vi "load config data.vi"(8 "error in (no error)":errorcluster, 11 "Sim Laser Driver in":refnum<class "Sim Laser Driver.lvclass">) -> (0 "error out":errorcluster, 3 "Sim Laser Driver out":refnum<class "Sim Laser Driver.lvclass">)   [LabVIEW 2022 SP3, in "Sim Laser Driver.lvclass"]
uses:
  Sim Laser Driver.lvclass
  C:/XY Stage/XY Stage/Framework/Base/Base.lvclass
  XY Stage/Framework/Base/Base.lvclass/Base.ctl
  Sim Laser Driver.lvclass/Sim Laser Driver.ctl
  c45f4fda-8063-4fab-8851-1de7a636a2c7.vi
  XY Stage/Framework/Base/Accessors/Read Config Path.vi
  XY Stage/Framework/Base/Accessors/Read Section.vi
  <vilib>/Utility/config.llb/Open Config Data.vi
  <userlib>/_OpenG.lib/variantconfig/variantconfig.llb/Read Section Cluster__ogtk.vi
  <vilib>/Utility/config.llb/Close Config Data.vi
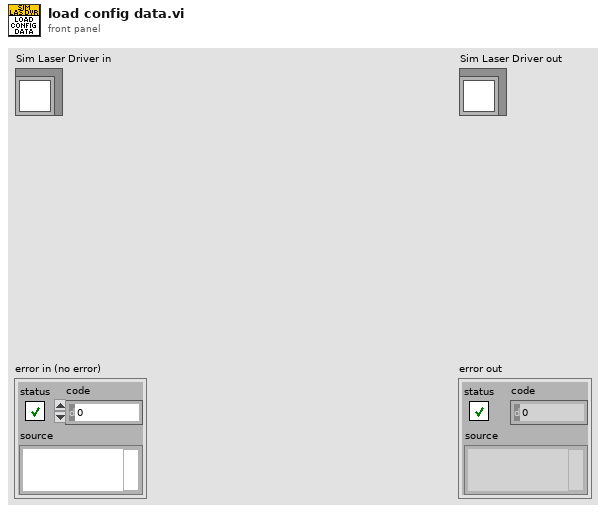
[diagram p1: front panel]
types:
  T1 = typedef "Sim Laser Driver.lvclass/settings.ctl" = cluster{"Power":dbl}
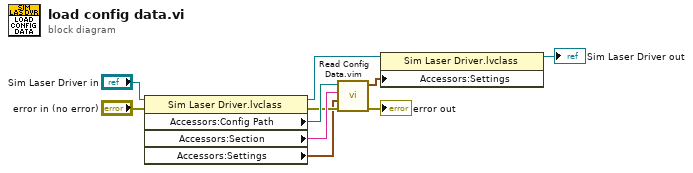
[diagram p0: block diagram]
diagram:
  n1 = property class="Sim Laser Driver.lvclass"(reference="Sim Laser Driver in", error in="error in (no error)") -> (reference out=w3:refnum<class "Sim Laser Driver.lvclass">, error out=w8:errorcluster, "Accessors:Config Path"=w10:path, "Accessors:Section"=w9:string, "Accessors:Settings"=w4:T1)
  n2 = call "Read Config Data.vim"("error in (no error)"=w8, "Section Formatted Cluster Type"=w4, "Section"=w9, "Config Path"=w10) -> ("error out"=→"error out":errorcluster, "Section Formatted Cluster Type 2"=w2:T1)  [unwired: 6 in]
  n3 = property class="Sim Laser Driver.lvclass"(reference=w3, "Accessors:Settings"=w2) -> (reference out=→"Sim Laser Driver out":refnum<class "Sim Laser Driver.lvclass">)  [unwired: 1 in, 1 out]
